vi "Main.vi"() -> ()   [LabVIEW 2019]
doc: "The Motion Sensor sample project uses the onboard accelerometer to detect motion and displays the amplitude by using the onboard LEDs of myRIO."
uses:
  Communication/TypeDef/#TypeDef_SetGet.ctl
  <vilib>/myRIO/Common/Instrument Driver Framework/myRIO v1.0/UART/vis/myRIO v1.0 Close UART.vi
  <vilib>/myRIO/Common/Instrument Driver Framework/Utilities/vis/FPGA Ref Manager.vi
  <vilib>/myRIO/Common/Instrument Driver Framework/myRIO v1.0/myRIO v1.0 Reset FPGA.vi
  <vilib>/myRIO/Common/Instrument Driver Framework/myRIO v1.0/IRQ/vis/myRIO v1.0 IRQ Info FGV.vi
  <vilib>/myRIO/Common/Instrument Driver Framework/myRIO v1.0/IRQ/vis/myRIO v1.0 Timer IRQ Info FGV.vi
  <vilib>/myRIO/Common/Instrument Driver Framework/myRIO v1.0/IRQ/vis/myRIO v1.0 ISR Agent.vi
  <vilib>/myRIO/Instrument Drivers/Utilities/vis/Reset Index.vi
  <vilib>/myRIO/Common/Instrument Driver Framework/myRIO v1.0/Resource Manager/vis/myRIO v1.0 Block Write Resource Manager.vi
  <vilib>/myRIO/Instrument Drivers/Utilities/Utilities.lvlib
panel:
  out "error out":errorcluster
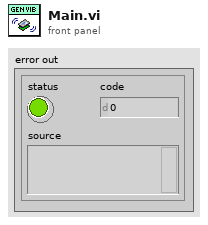
[diagram p1: front panel]
types:
  T1 = typedef "#TypeDef_SetGet.ctl" = enum16{"Set", "Get"}
  T2 = typedef "#TypeDef_MyRIO_Queues.ctl" = cluster{"FromDAtoDP":refnum<queue>, "FromMyRIOtoPC":refnum<k21>, "FromPCtoMyRIO":refnum<k21>}
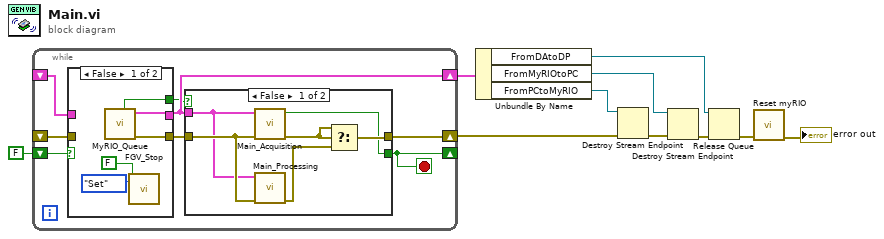
[diagram p0: block diagram]
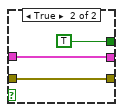
[diagram p2: hidden frame]
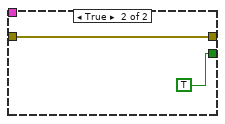
[diagram p3: hidden frame]
diagram:
  n1 = while {
    shift-right: [w17] -> w9
    shift-left: _ -> [w14]
    shift-right: [w11] -> _
    shift-left: FALSE ("Stop") -> [w13]
    shift-right: [w16] -> w8
    shift-left: _ -> [w12]
    stop <- w11 stop-if-true
    n2 = case shown="False" w13 {
      tunnel: [w23 w26] -> w18
      tunnel: [w22 w24] -> w16
      tunnel: [w21 TRUE ("Error Conneciton")] -> w15
      tunnel: w14 -> [_ w26]
      tunnel: w12 -> [_ w24]
      frame False {
        n3 = call "MyRIO_Queue.vi"() -> ("error out"=w23:errorcluster, "Queues out"=w22:T2, "Error Conneciton"=w21:bool)  [unwired: 9 in]
        n4 = call "FGV_Stop.vi"("Get/Set"=#TypeDef_SetGet."Set", "STOP in"=FALSE) -> ()  [unwired: 9 in, 1 out]
      }
      frame True {
      }
    }
    n5 = case shown="False" w15 {
      tunnel: w18 -> [w32 w33]
      tunnel: [w27 TRUE ("Stop")] -> w11
      tunnel: [w29 w33] -> w17
      tunnel: w16 -> [w28 _]
      frame False {
        n6 = call "Main_Acquisition.vi"("error in"=w32, "Queues in"=w28) -> ("error out"=w31:errorcluster, "Stop?"=w27:bool)  [unwired: 8 in]
        n7 = call "Main_Processing.vi"("error in"=w32, "Queues in"=w28) -> ("error out"=w30:errorcluster)  [unwired: 9 in]
        n8 = Select(t=w31, s=w31, f=w30) -> (s? t:f=w29:errorcluster)
      }
      frame True {
      }
    }
  }
  n9 = Unbundle By Name(w8) -> ("FromDAtoDP"=w7:refnum<queue>, "FromMyRIOtoPC"=w6:refnum<k21>, "FromPCtoMyRIO"=w5:refnum<k21>)
  n10 = Destroy Stream Endpoint(8:w9, 11:w5) -> (0:w10:errorcluster)
  n11 = Destroy Stream Endpoint(8:w10, 11:w6) -> (0:w4:errorcluster)
  n12 = Release Queue(queue=w7, error in (no error)=w4) -> (error out=w2:errorcluster)  [unwired: 1 in, 2 out]
  n13 = call <vilib>:"Reset myRIO.vi"("error in (no error)"=w2) -> ("error out"=→"error out":errorcluster)  [unwired: 10 in]
